vi "Climb.vi"() -> ()   [LabVIEW 2013]
uses:
  Robot Global Data.vi
  ClimbStates.ctl
  <vilib>/Rock Robotics/SystemInterfaces/DIO/FPGA_DIOChannel.ctl
  <vilib>/Rock Robotics/SystemInterfaces/Typedef/FPGA_TypedefDigitalModule.ctl
  <vilib>/Rock Robotics/WPI/DigitalInput/WPI_DigitalInputDevRef.ctl
panel:
  out "Shooter":bool
  out "HooksMiddle":bool
  out "HooksIn":bool
  out "HooksOut":bool
  out "ArmMiddle":bool
  out "ArmInOut":bool
  out "ResumeState":T1
  out "CommandState":T1
  in  "CurrentCount2":i32
  in  "CurrentCount":i32
  in  "input cluster":T5={"ArmInOut"={"DevStatus"={"status"=FALSE, "code"=0, "source"=""}, "DIO Channel"=enum."Invalid", "Digital Module"=enum."Digital Module 1"}, "ArmMiddle"={"DevStatus"={"status"=FALSE, "code"=0, "source"=""}, "DIO Channel"=enum."Invalid", "Digital Module"=enum."Digital Module 1"}, "HooksOut"={"DevStatus"={"status"=FALSE, "code"=0, "source"=""}, "DIO Channel"=enum."Invalid", "Digital Module"=enum."Digital Module 1"}, "HooksIn"={"DevStatus"={"status"=FALSE, "code"=0, "source"=""}, "DIO Channel"=enum."Invalid", "Digital Module"=enum."Digital Module 1"}, "HooksMiddle"={"DevStatus"={"status"=FALSE, "code"=0, "source"=""}, "DIO Channel"=enum."Invalid", "Digital Module"=enum."Digital Module 1"}, "Shooter"={"DevStatus"={"status"=FALSE, "code"=0, "source"=""}, "DIO Channel"=enum."Invalid", "Digital Module"=enum."Digital Module 1"}}
  # "BE SURE THESE DEFAULT TO 0!!!"
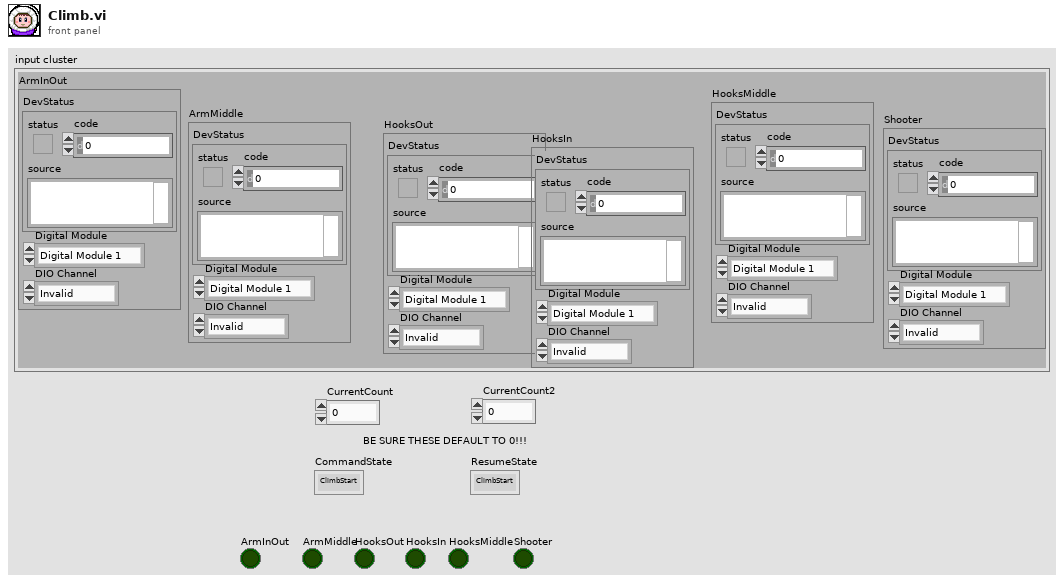
[diagram p1: front panel]
types:
  T1 = typedef "ClimbStates.ctl" = enum16{"ClimbStart", "DriveBack", "ActivateHooks", "ArmExtends", "Rachet re-engage", "Arm 60deg", "PullRobot", "Setdown", "Arm Extend2", "Rachet re-engage2", "Arm60deg2", "PullRobot2", "Setdown2", "Arm Extend3", "Rachet re-engage3", "Arm 60deg3", "Pullrobot3", "Pause"}
  T2 = typedef "WPI_DigitalInputDevRef.ctl" = cluster{"DevStatus":errorcluster, "DIO Channel":T3, "Digital Module":T4}
  T3 = typedef "FPGA_DIOChannel.ctl" = enum8{"DIO 1", "DIO 2", "DIO 3", "DIO 4", "DIO 5", "DIO 6", "DIO 7", "DIO 8", "DIO 9", "DIO 10", "DIO 11", "DIO 12", "DIO 13", "DIO 14", "Invalid"}
  T4 = typedef "FPGA_TypedefDigitalModule.ctl" = enum16{"Digital Module 1", "Digital Module 2"}
  T5 = cluster{"ArmInOut":T2, "ArmMiddle":T2, "HooksOut":T2, "HooksIn":T2, "HooksMiddle":T2, "Shooter":T2}
  T6 = typedef "LoopDisable.ctl" = cluster{"Climb.vi":bool, "LauncherAngle.vi":bool, "Launcher.vi":bool, "ArmControl.vi":bool, "WinchMotor.vi":bool, "ReadDriveEncoder.vi":bool}
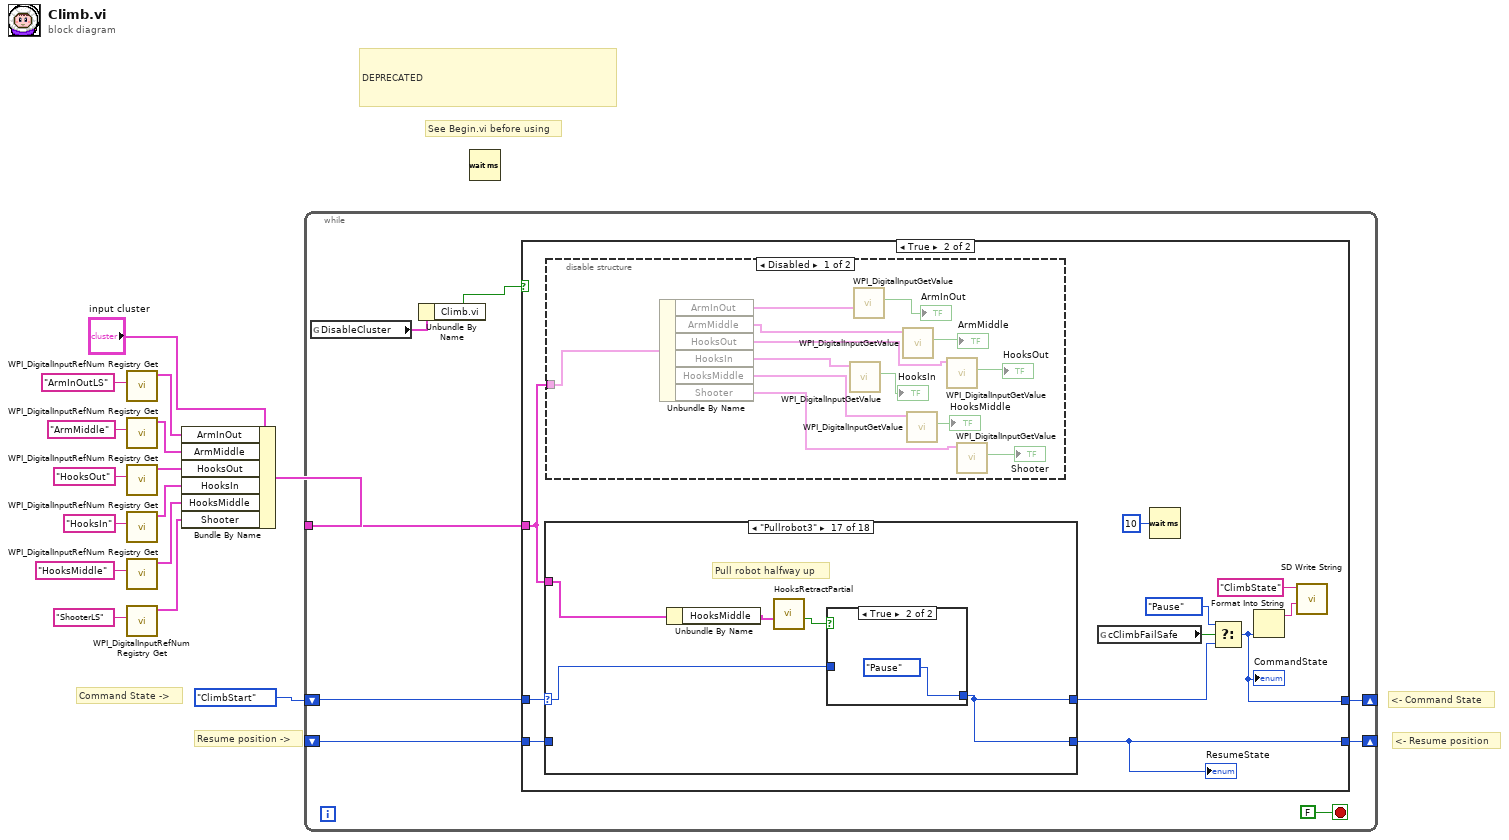
[diagram p0: block diagram]
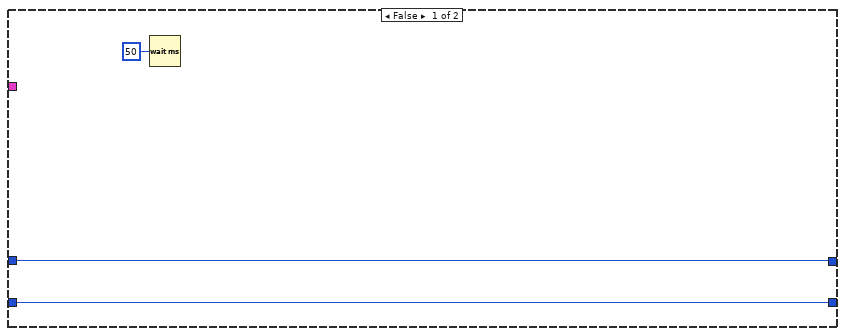
[diagram p2: hidden frame]
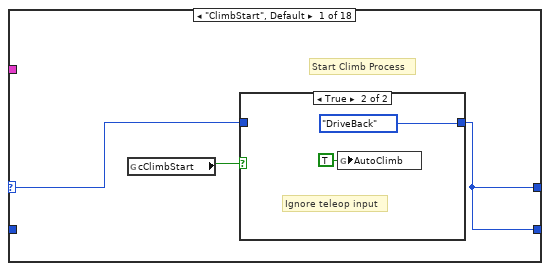
[diagram p4: hidden frame]
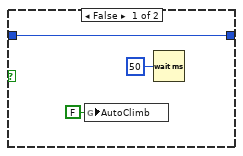
[diagram p5: hidden frame]
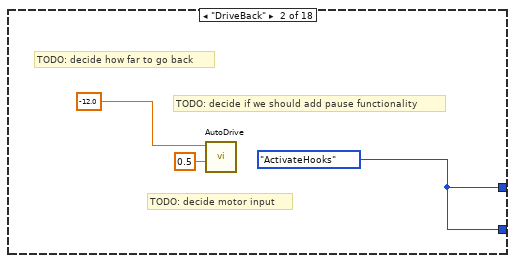
[diagram p6: hidden frame]
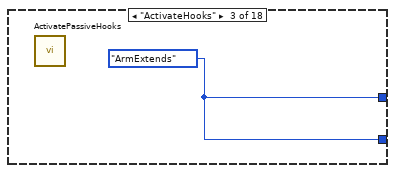
[diagram p7: hidden frame]
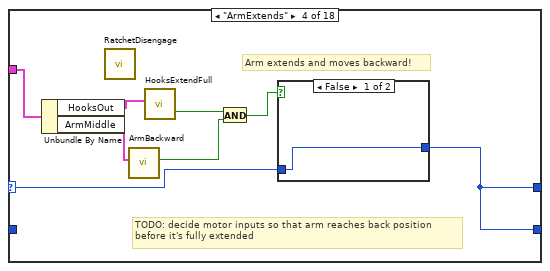
[diagram p8: hidden frame]
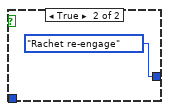
[diagram p9: hidden frame]
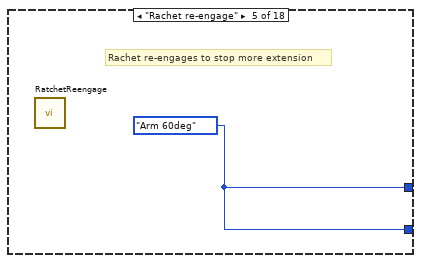
[diagram p10: hidden frame]
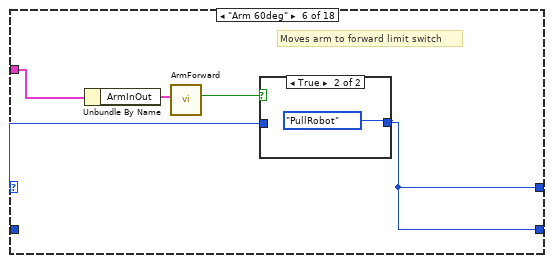
[diagram p11: hidden frame]
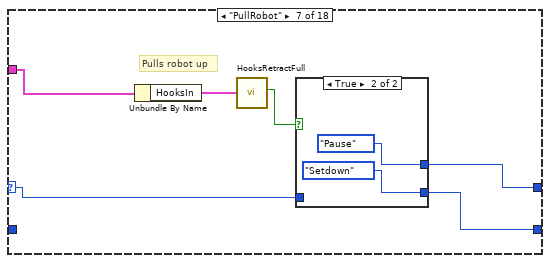
[diagram p13: hidden frame]
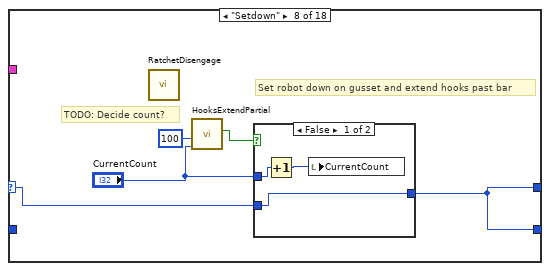
[diagram p15: hidden frame]
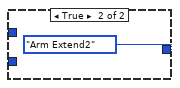
[diagram p16: hidden frame]
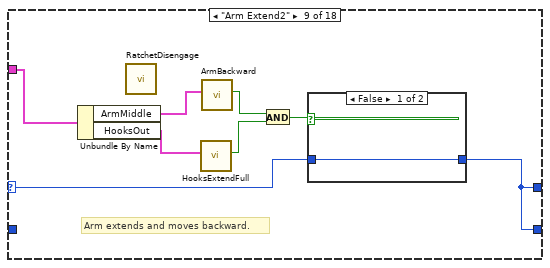
[diagram p17: hidden frame]
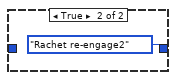
[diagram p18: hidden frame]
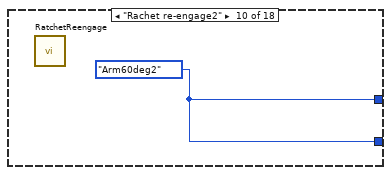
[diagram p19: hidden frame]
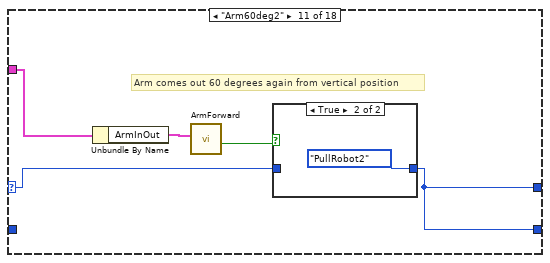
[diagram p20: hidden frame]
diagram:
  # "See Begin.vi before using"
  # "DEPRECATED"
  # "Resume position ->"
  # "Command State ->"
  # "<- Resume position"
  # "<- Command State"
  n1 = call <vilib>:"WPI_DigitalInputRefNum Registry Get.vi"("refnum name"="ArmInOutLS") -> ("DigitalInputDevRef"=w8:T2)  [unwired: 9 in, 1 out]
  n2 = call <vilib>:"WPI_DigitalInputRefNum Registry Get.vi"("refnum name"="ArmMiddle") -> ("DigitalInputDevRef"=w6:T2)  [unwired: 9 in, 1 out]
  n3 = call <vilib>:"WPI_DigitalInputRefNum Registry Get.vi"("refnum name"="HooksOut") -> ("DigitalInputDevRef"=w5:T2)  [unwired: 9 in, 1 out]
  n4 = call <vilib>:"WPI_DigitalInputRefNum Registry Get.vi"("refnum name"="HooksIn") -> ("DigitalInputDevRef"=w4:T2)  [unwired: 9 in, 1 out]
  n5 = call <vilib>:"WPI_DigitalInputRefNum Registry Get.vi"("refnum name"="HooksMiddle") -> ("DigitalInputDevRef"=w3:T2)  [unwired: 9 in, 1 out]
  n6 = call <vilib>:"WPI_DigitalInputRefNum Registry Get.vi"("refnum name"="ShooterLS") -> ("DigitalInputDevRef"=w2:T2)  [unwired: 9 in, 1 out]
  n7 = Bundle By Name(cluster="input cluster", "ArmInOut"=w8, "ArmMiddle"=w6, "HooksOut"=w5, "HooksIn"=w4, "HooksMiddle"=w3, "Shooter"=w2) -> (w1:T5)
  n8 = while {
    shift-right: [w19] -> _
    shift-left: ClimbStates."ClimbStart" -> [w22]
    shift-right: [w20] -> _
    shift-left: _ -> [w21]
    tunnel: w1 -> [w18]
    stop <- FALSE stop-if-true
    n9 = global read "Robot Global Data.vi" "DisableCluster"() -> (w17:T6)
    n10 = Unbundle By Name(w17) -> ("Climb.vi"=w16:bool)
    n11 = case shown="True" w16 {
      tunnel: w22 -> [w26 w37]
      tunnel: w21 -> [w25 w34]
      tunnel: [w25 w33] -> w20
      tunnel: [w26 w30] -> w19
      tunnel: w18 -> [_ w27]
      frame False {
        n12 = Wait (ms)(milliseconds to wait=u32 50) -> ()  [unwired: 1 out]
      }
      frame True {
        n13 = case shown="\"Pullrobot3\"" w37 {
          selector: w37 -> [w52 _ _ w68 _ w75 w83 w93 w104 _ w111 w120 w129 w140 _ w147 w156 _]
          tunnel: [w51 w59 w62 w67 w73 w74 w82 w92 w103 w109 w110 w118 w128 w139 w145 w146 w155 w161] -> w35
          tunnel: w34 -> [_ _ _ _ _ _ _ _ _ _ _ _ _ _ _ _ _ w163]
          tunnel: [w51 w59 w62 w67 w73 w74 w81 w92 w103 w109 w110 w117 w128 w139 w145 w146 w155 w163] -> w33
          tunnel: w27 -> [_ _ _ w70 _ w78 w86 _ w105 _ w112 w119 _ w141 _ w148 w154 _]
          frame "ClimbStart", Default {
            # "Start Climb Process"
            n14 = global read "Robot Global Data.vi" "cClimbStart"() -> (w53:bool)
            n15 = case shown="True" w53 {
              tunnel: [w56 ClimbStates."DriveBack"] -> w51
              tunnel: w52 -> [w56 _]
              frame False {
                n16 = global write "Robot Global Data.vi" "AutoClimb"(FALSE ("AutoClimb")) -> ()
                n17 = Wait (ms)(milliseconds to wait=u32 50) -> ()  [unwired: 1 out]
              }
              frame True {
                # "Ignore teleop input"
                n18 = global write "Robot Global Data.vi" "AutoClimb"(TRUE ("AutoClimb")) -> ()
              }
            }
          }
          frame "DriveBack" {
            w59 = ClimbStates."ActivateHooks"
            # "TODO: decide if we should add pause functionality"
            # "TODO: decide motor input"
            # "TODO: decide how far to go back"
            n19 = call "AutoDrive.vi"("Steady Val"=0.5, "Distance to travel (inches)"=-12.0) -> ()  [unwired: 10 in]
          }
          frame "ActivateHooks" {
            w62 = ClimbStates."ArmExtends"
            n20 = call "ActivatePassiveHooks.vi"() -> ()  [unwired: 12 in]
          }
          frame "ArmExtends" {
            # "TODO: decide motor inputs so that arm reaches back position\nbefore it's fully extended"
            # "Arm extends and moves backward!"
            n21 = Unbundle By Name(w70) -> ("HooksOut"=w69:T2, "ArmMiddle"=w66:T2)
            n22 = call "RatchetDisengage.vi"() -> ()  [unwired: 12 in]
            n23 = call "ArmBackward.vi"("BackwardLimitSwitch"=w66) -> ("Done?"=w64:bool)  [unwired: 10 in]
            n24 = call "HooksExtendFull.vi"("HooksOutLimitSwitch"=w69) -> ("Done?"=w65:bool)  [unwired: 10 in]
            n25 = And(x=w65, y=w64) -> (x .and. y?=w63:bool)
            n26 = case shown="False" w63 {
              tunnel: w68 -> [w71 _]
              tunnel: [w71 ClimbStates."Rachet re-engage"] -> w67
              frame False {
              }
              frame True {
              }
            }
          }
          frame "Rachet re-engage" {
            w73 = ClimbStates."Arm 60deg"
            # "Rachet re-engages to stop more extension"
            n27 = call "RatchetReengage.vi"() -> ()  [unwired: 12 in]
          }
          frame "Arm 60deg" {
            # "Moves arm to forward limit switch"
            n28 = Unbundle By Name(w78) -> ("ArmInOut"=w77:T2)
            n29 = call "ArmForward.vi"("ForwardLimitSwitch"=w77) -> ("Done?"=w76:bool)  [unwired: 10 in]
            n30 = case shown="True" w76 {
              tunnel: w75 -> [w79 _]
              tunnel: [w79 ClimbStates."PullRobot"] -> w74
              frame False {
              }
              frame True {
              }
            }
          }
          frame "PullRobot" {
            # "Pulls robot up"
            n31 = Unbundle By Name(w86) -> ("HooksIn"=w85:T2)
            n32 = call "HooksRetractFull.vi"("HooksInLimitSwitch"=w85) -> ("Done?"=w84:bool)  [unwired: 10 in]
            n33 = case shown="True" w84 {
              tunnel: w83 -> [w87 _]
              tunnel: [w87 ClimbStates."Setdown"] -> w81
              tunnel: [w87 ClimbStates."Pause"] -> w82
              frame False {
              }
              frame True {
              }
            }
          }
          frame "Setdown" {
            # "TODO: Decide count?"
            # "Set robot down on gusset and extend hooks past bar"
            n34 = call "RatchetDisengage.vi"() -> ()  [unwired: 12 in]
            n35 = call "HooksExtendPartial.vi"("CurrentCount"="CurrentCount", "DesiredCount"=100) -> ("Done?"=w94:bool)  [unwired: 9 in]
            n36 = case shown="False" w94 {
              tunnel: w93 -> [w97 _]
              tunnel: [w97 ClimbStates."Arm Extend2"] -> w92
              tunnel: "CurrentCount" -> [w96 _]
              frame False {
                n37 = Increment(x=w96) -> (x+1=w95:i32)
                n38 = local write "CurrentCount"(w95) -> ()
              }
              frame True {
              }
            }
          }
          frame "Arm Extend2" {
            # "Arm extends and moves backward."
            n39 = Unbundle By Name(w105) -> ("ArmMiddle"=w102:T2, "HooksOut"=w106:T2)
            n40 = call "RatchetDisengage.vi"() -> ()  [unwired: 12 in]
            n41 = call "HooksExtendFull.vi"("HooksOutLimitSwitch"=w106) -> ("Done?"=w100:bool)  [unwired: 10 in]
            n42 = call "ArmBackward.vi"("BackwardLimitSwitch"=w102) -> ("Done?"=w101:bool)  [unwired: 10 in]
            n43 = And(x=w101, y=w100) -> (x .and. y?=w99:bool)
            n44 = case shown="False" w99 {
              tunnel: w104 -> [w107 _]
              tunnel: [w107 ClimbStates."Rachet re-engage2"] -> w103
              frame False {
              }
              frame True {
              }
            }
          }
          frame "Rachet re-engage2" {
            w109 = ClimbStates."Arm60deg2"
            n45 = call "RatchetReengage.vi"() -> ()  [unwired: 12 in]
          }
          frame "Arm60deg2" {
            # "Arm comes out 60 degrees again from vertical position"
            n46 = Unbundle By Name(w112) -> ("ArmInOut"=w114:T2)
            n47 = call "ArmForward.vi"("ForwardLimitSwitch"=w114) -> ("Done?"=w113:bool)  [unwired: 10 in]
            n48 = case shown="True" w113 {
              tunnel: w111 -> [w115 _]
              tunnel: [w115 ClimbStates."PullRobot2"] -> w110
              frame False {
              }
              frame True {
              }
            }
          }
          frame "PullRobot2" {
            # "Pulls robot up"
            n49 = Unbundle By Name(w119) -> ("HooksIn"=w122:T2)
            n50 = call "HooksRetractFull.vi"("HooksInLimitSwitch"=w122) -> ("Done?"=w121:bool)  [unwired: 10 in]
            n51 = case shown="True" w121 {
              tunnel: w120 -> [w123 _]
              tunnel: [w123 ClimbStates."Setdown2"] -> w117
              tunnel: [w123 ClimbStates."Pause"] -> w118
              frame False {
              }
              frame True {
              }
            }
          }
          frame "Setdown2" {
            # "TODO: Decide count?"
            # "Set robot down on gusset (should be on 2nd level now)  and extend hooks past bar"
            n52 = call "RatchetDisengage.vi"() -> ()  [unwired: 12 in]
            n53 = call "HooksExtendPartial.vi"("CurrentCount"="CurrentCount2", "DesiredCount"=100) -> ("Done?"=w130:bool)  [unwired: 9 in]
            n54 = case shown="True" w130 {
              tunnel: w129 -> [w133 _]
              tunnel: [w133 ClimbStates."Arm Extend3"] -> w128
              tunnel: "CurrentCount2" -> [w132 _]
              frame False {
                n55 = Increment(x=w132) -> (x+1=w131:i32)
                n56 = local write "CurrentCount2"(w131) -> ()
              }
              frame True {
              }
            }
          }
          frame "Arm Extend3" {
            # "Arm extends and moves back!"
            n57 = call "RatchetDisengage.vi"() -> ()  [unwired: 12 in]
            n58 = Unbundle By Name(w141) -> ("ArmMiddle"=w138:T2, "HooksOut"=w142:T2)
            n59 = call "ArmBackward.vi"("BackwardLimitSwitch"=w138) -> ("Done?"=w137:bool)  [unwired: 10 in]
            n60 = call "HooksExtendFull.vi"("HooksOutLimitSwitch"=w142) -> ("Done?"=w136:bool)  [unwired: 10 in]
            n61 = And(x=w137, y=w136) -> (x .and. y?=w135:bool)
            n62 = case shown="True" w135 {
              tunnel: w140 -> [w143 _]
              tunnel: [w143 ClimbStates."Rachet re-engage3"] -> w139
              frame False {
              }
              frame True {
              }
            }
          }
          frame "Rachet re-engage3" {
            w145 = ClimbStates."Arm 60deg3"
            n63 = call "RatchetReengage.vi"() -> ()  [unwired: 12 in]
          }
          frame "Arm 60deg3" {
            # "Arm comes out 60 degrees again from vertical position"
            n64 = Unbundle By Name(w148) -> ("ArmInOut"=w150:T2)
            n65 = call "ArmForward.vi"("ForwardLimitSwitch"=w150) -> ("Done?"=w149:bool)  [unwired: 10 in]
            n66 = case shown="True" w149 {
              tunnel: w147 -> [w151 _]
              tunnel: [w151 ClimbStates."Pullrobot3"] -> w146
              frame False {
              }
              frame True {
              }
            }
          }
          frame "Pullrobot3" {
            # "Pull robot halfway up"
            n67 = Unbundle By Name(w154) -> ("HooksMiddle"=w153:T2)
            n68 = call "HooksRetractPartial.vi"("HooksMiddleLimitSwitch"=w153) -> ("Done?"=w157:bool)  [unwired: 10 in]
            n69 = case shown="True" w157 {
              tunnel: w156 -> [w158 _]
              tunnel: [w158 ClimbStates."Pause"] -> w155
              frame False {
              }
              frame True {
              }
            }
          }
          frame "Pause" {
            # "Pauses the robot"
            n70 = global read "Robot Global Data.vi" "cClimbResume"() -> (w164:bool)
            n71 = case shown="False" w164 {
              tunnel: w163 -> [_ w171]
              tunnel: [ClimbStates."Pause" w171] -> w160
              frame False {
                n72 = global write "Robot Global Data.vi" "AutoClimb"(FALSE ("AutoClimb")) -> ()
                n73 = call "RatchetReengage.vi"() -> ()  [unwired: 12 in]
                n74 = Wait (ms)(milliseconds to wait=u32 50) -> ()  [unwired: 1 out]
              }
              frame True {
                n75 = global write "Robot Global Data.vi" "AutoClimb"(TRUE ("AutoClimb")) -> ()
              }
            }
            n76 = global read "Robot Global Data.vi" "cClimbReset"() -> (w162:bool)
            n77 = case shown="True" w162 {
              tunnel: [w165 ClimbStates."ClimbStart"] -> w161
              tunnel: w160 -> [w165 _]
              frame False {
              }
              frame True {
              }
            }
          }
        }
        "ResumeState" <- w33
        n78 = disable-structure shown="Disabled" {
          disable-tunnel: w27 -> [w50 _]
          frame Disabled {
            n79 = Unbundle By Name(w50) -> ("ArmInOut"=w49:T2, "ArmMiddle"=w47:T2, "HooksOut"=w45:T2, "HooksIn"=w43:T2, "HooksMiddle"=w41:T2, "Shooter"=w39:T2)
            n80 = call <vilib>:"WPI_DigitalInputGetValue.vi"("DigitalInputDevRef"=w43) -> ("Value"=→"HooksIn":bool)  [unwired: 8 in, 2 out]
            n81 = call <vilib>:"WPI_DigitalInputGetValue.vi"("DigitalInputDevRef"=w49) -> ("Value"=→"ArmInOut":bool)  [unwired: 8 in, 2 out]
            n82 = call <vilib>:"WPI_DigitalInputGetValue.vi"("DigitalInputDevRef"=w47) -> ("Value"=→"ArmMiddle":bool)  [unwired: 8 in, 2 out]
            n83 = call <vilib>:"WPI_DigitalInputGetValue.vi"("DigitalInputDevRef"=w41) -> ("Value"=→"HooksMiddle":bool)  [unwired: 8 in, 2 out]
            n84 = call <vilib>:"WPI_DigitalInputGetValue.vi"("DigitalInputDevRef"=w45) -> ("Value"=→"HooksOut":bool)  [unwired: 8 in, 2 out]
            n85 = call <vilib>:"WPI_DigitalInputGetValue.vi"("DigitalInputDevRef"=w39) -> ("Value"=→"Shooter":bool)  [unwired: 8 in, 2 out]
          }
          frame Enabled {
          }
        }
        n86 = global read "Robot Global Data.vi" "cClimbFailSafe"() -> (w36:bool)
        n87 = Wait (ms)(milliseconds to wait=u32 10) -> ()  [unwired: 1 out]
        n88 = Select(t=ClimbStates."Pause", s=w36, f=w35) -> (s? t:f=w30:T1)
        "CommandState" <- w30
        n89 = Format Into String(w30) -> (resulting string=w29:string)  [unwired: 3 in, 1 out]
        n90 = call <vilib>:"SD Write String.vi"("String"=w29, "Name"="ClimbState") -> ()  [unwired: 8 in, 2 out]
      }
    }
  }
  n91 = Wait (ms)() -> ()  [unwired: 1 in, 1 out]
